vi "Update Layout.vi"(8 "error in (no error)":errorcluster, 10 "UI Refs":T1, 11 "ArrayManager in":refnum<class "ArrayManager.lvclass">) -> (0 "error out":errorcluster, 3 "ArrayManager out":refnum<class "ArrayManager.lvclass">)   [LabVIEW 2020, in "OOPanel.lvlib" / "ArrayManager.lvclass"]
uses:
  ArrayManager.lvclass
  UI Refs.ctl
  ArrayManager.lvclass/ArrayManager.ctl
  ArrayPanel/ArrayPanel.lvclass
  C:/dev/lv20CE/lv-oopanel/OOPanel/Panel/Panel.lvclass
  Manager/Manager.lvclass
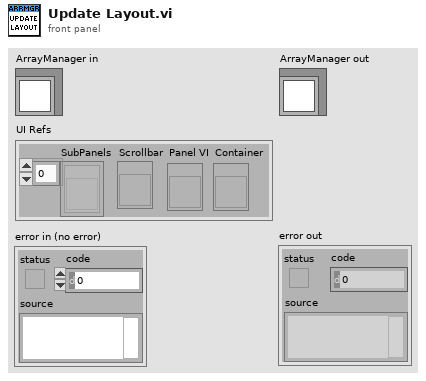
[diagram p1: front panel]
types:
  T1 = typedef "OOPanel.lvlib/ArrayManager.lvclass/UI Refs.ctl" = cluster{"SubPanels":refnum<vi>[], "Scrollbar":refnum<vi>, "Panel VI":refnum<vi>, "Container":refnum<vi>}
  T2 = typedef "OOPanel.lvlib/Desired Size.ctl" = cluster{"Width":u32, "Height":u32}
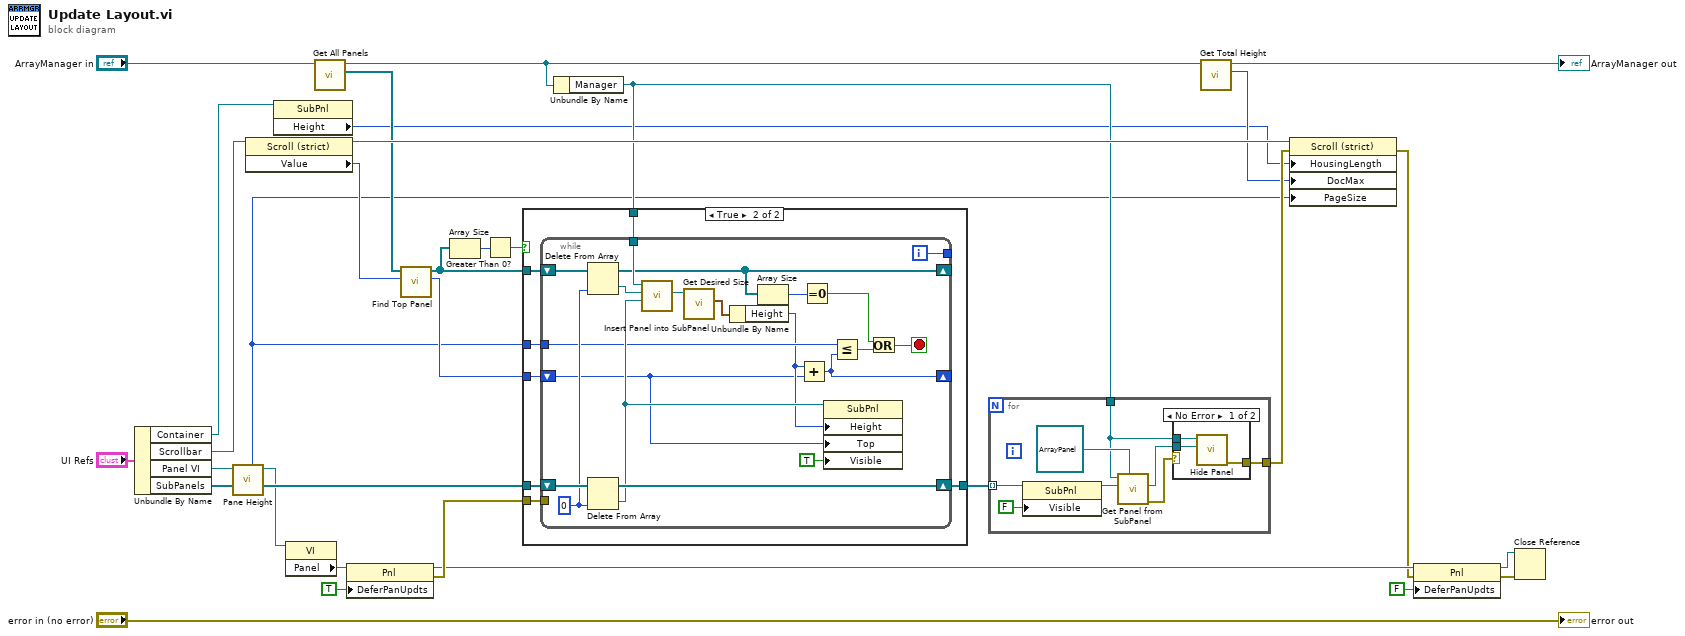
[diagram p0: block diagram]
diagram:
  n1 = Unbundle By Name("UI Refs") -> ("Container"=w2:refnum<vi>, "Scrollbar"=w28:refnum<vi>, "Panel VI"=w25:refnum<vi>, "SubPanels"=w26:refnum<vi>[])
  n2 = call "Pane Height.vi"("Panel VI in"=w25) -> ("Panel VI"=w24:refnum<vi>, "Height"=w6:u32)  [unwired: 9 in]
  n3 = property class="Scroll (strict)"(reference=w28) -> (reference out=w27:refnum<vi>, "Value"=w8:i32)  [unwired: 1 in, 1 out]
  n4 = property class="SubPnl"(reference=w2) -> ("Height"=w1:u32)  [unwired: 1 in, 2 out]
  n5 = property class="VI"(reference=w24) -> ("Panel"=w23:refnum<vi>)  [unwired: 1 in, 2 out]
  n6 = call "Get All Panels.vi"("PanelArray in"="ArrayManager in") -> ("Panels"=w9:refnum<class "ArrayPanel.lvclass">[], "PanelArray out"=w12:refnum<class "ArrayManager.lvclass">)  [unwired: 8 in, 1 out]
  n7 = property class="Pnl"(reference=w23, "DeferPanUpdts"=TRUE ("Defer Panel Updates")) -> (reference out=w19:refnum<vi>, error out=w21:errorcluster)  [unwired: 1 in]
  n8 = call "Find Top Panel.vi"("Scroll"=w8, "All Panels"=w9) -> ("Start"=w7:i32, "Panels"=w5:refnum<class "ArrayPanel.lvclass">[])  [unwired: 8 in]
  n9 = Array Size(array=w5) -> (size(s)=w4:i32)
  n10 = Greater Than 0?(x=w4) -> (x > 0?=w3:bool)
  n11 = Unbundle By Name(w12) -> ("Manager"=w13:refnum<class "Manager.lvclass">)
  n12 = case shown="True" w3 {
    tunnel: w26 -> [w32 w39]
    tunnel: w21 -> [_ w38]
    tunnel: [w32 w37] -> w14
    tunnel: w13 -> [_ w36]
    tunnel: w7 -> [_ w35]
    tunnel: w6 -> [_ w34]
    tunnel: w5 -> [_ w33]
    frame False {
    }
    frame True {
      n13 = while {
        shift-right: [w58] -> w37
        shift-left: w39 -> [w59]
        tunnel: w34 -> [w49]
        tunnel: w38 -> [_]
        shift-right: [w45] -> _
        shift-left: w33 -> [w57]
        tunnel: w36 -> [w55]
        shift-right: [w48] -> _
        shift-left: w35 -> [w40]
        tunnel: [w46] -> _
        i -> [w46]
        stop <- w43 stop-if-true
        w56 = 0 ("index")
        n14 = Delete From Array(array=w57, index=w56) -> (deleted portion=w54:refnum<class "ArrayPanel.lvclass">, array with subset deleted=w45:refnum<class "ArrayPanel.lvclass">[])  [unwired: 1 in]
        n15 = Delete From Array(array=w59, index=w56) -> (deleted portion=w53:refnum<vi>, array with subset deleted=w58:refnum<vi>[])  [unwired: 1 in]
        n16 = call "Insert Panel into SubPanel.vi"("SubPanel"=w53, "Panel In"=w54, "Manager in"=w55) -> ("Panel"=w51:refnum<class "ArrayPanel.lvclass">)  [unwired: 6 in, 2 out]
        n17 = call-dynamic "Get Desired Size.vi"("ArrayPanel in"=w51) -> ("Desired Size"=w50:T2)  [unwired: 8 in, 2 out]
        n18 = Unbundle By Name(w50) -> ("Height"=w41:u32)
        n19 = Array Size(array=w45) -> (size(s)=w44:i32)
        n20 = Add(x=w41, y=w40) -> (x+y=w48:u32)
        n21 = Equal To 0?(x=w44) -> (x = 0?=w42:bool)
        n22 = property class="SubPnl"(reference=w53, "Height"=w41, "Top"=w40, "Visible"=TRUE) -> ()  [unwired: 1 in, 2 out]
        n23 = Less Or Equal?(x=w49, y=w48) -> (x <= y?=w47:bool)
        n24 = Or(x=w42, y=w47) -> (x .or. y?=w43:bool)
      }
    }
  }
  n25 = for {
    tunnel: w14 -> [w63] mode=indexing
    tunnel: w13 -> [w64]
    tunnel: [w60] -> w31
    n26 = property class="SubPnl"(reference=w63, "Visible"=FALSE) -> (reference out=w62:refnum<vi>)  [unwired: 1 in, 1 out]
    n27 = call "Get Panel from SubPanel.vi"("Panel Type (Panel)"=refnum<class "ArrayPanel.lvclass"> refnum ("OOPanel.lvlib:ArrayPanel.lvclass"), "SubPanel"=w62, "Manager in"=w64) -> ("error out"=w66:errorcluster, "Panel"=w65:refnum<class "ArrayPanel.lvclass">)  [unwired: 5 in, 2 out]
    n28 = case shown="No Error" w66 {
      tunnel: w65 -> [w70 _]
      tunnel: w64 -> [w69 _]
      tunnel: [w68 _] -> w60
      frame No Error {
        n29 = call "Hide Panel.vi"("Panel In"=w70, "Manager in"=w69) -> ("error out"=w68:errorcluster)  [unwired: 7 in, 2 out]
      }
      frame Error {
      }
    }
  }
  n30 = call "Get Total Height.vi"("ArrayManager in"=w12) -> ("Total Height"=w10:u32, "ArrayManager out"=→"ArrayManager out":refnum<class "ArrayManager.lvclass">)  [unwired: 8 in, 1 out]
  n31 = property class="Scroll (strict)"(reference=w27, error in=w31, "HousingLength"=w1, "DocMax"=w10, "PageSize"=w6) -> (error out=w17:errorcluster)  [unwired: 1 out]
  n32 = property class="Pnl"(reference=w19, error in=w17, "DeferPanUpdts"=FALSE ("Defer Panel Updates")) -> (reference out=w15:refnum<vi>, error out=w16:errorcluster)
  n33 = Close Reference(reference=w15, error in (no error)=w16) -> ()  [unwired: 1 out]
  "error out" <- "error in (no error)"
